vi "append time stamp.vi"(11 "Error in":refnum<class>) -> (3 "Error out":refnum<class "Error.lvclass">)   [LabVIEW 2020, in "Error Interface.lvlib" / "Error.lvclass"]
doc: "Appends current timestamp to the object private data"
uses:
  Error.lvclass
  Error.lvclass/Error.ctl
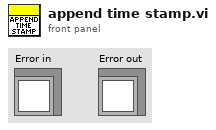
[diagram p1: front panel]
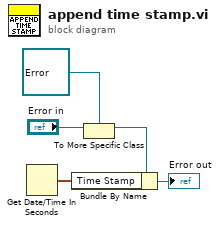
[diagram p0: block diagram]
diagram:
  n1 = Get Date/Time In Seconds() -> (seconds since 1Jan1904=w1:timestamp)
  n2 = To More Specific Class(target class=refnum<class "Error.lvclass"> refnum ("Error in 2"), reference="Error in") -> (specific class reference=w3:refnum<class "Error.lvclass">)  [unwired: 1 in, 1 out]
  n3 = Bundle By Name(cluster=w3, "Time Stamp"=w1) -> (→"Error out":refnum<class "Error.lvclass">)
